vi "Questao1VF_Ulisses.vi"() -> ()   [LabVIEW 2019]
uses:
  <vilib>/measure/matone.llb/Extract Multiple Tone Information 1 Chan.vi
  <vilib>/measure/NI_MAPro.lvlib
panel:
  out "Atende?":bool
  out "DHT(%)":dbl
  out "Fundamental":dbl
  out "Raiz":dbl
  out "Soma Quadratica":dbl
  in  "stop":bool
  in  "LIGAR":bool
  in  "file path":path=path "C:/lista2.tdms"
  out "ONDA COMPLETA":waveform(dbl)(graph)
  out "informação das ondas":T1(array[cluster]) {"detected phase (deg)" format="%_6g"; "detected amplitude" format="%_6p"; "detected frequency" format="%_6p"}
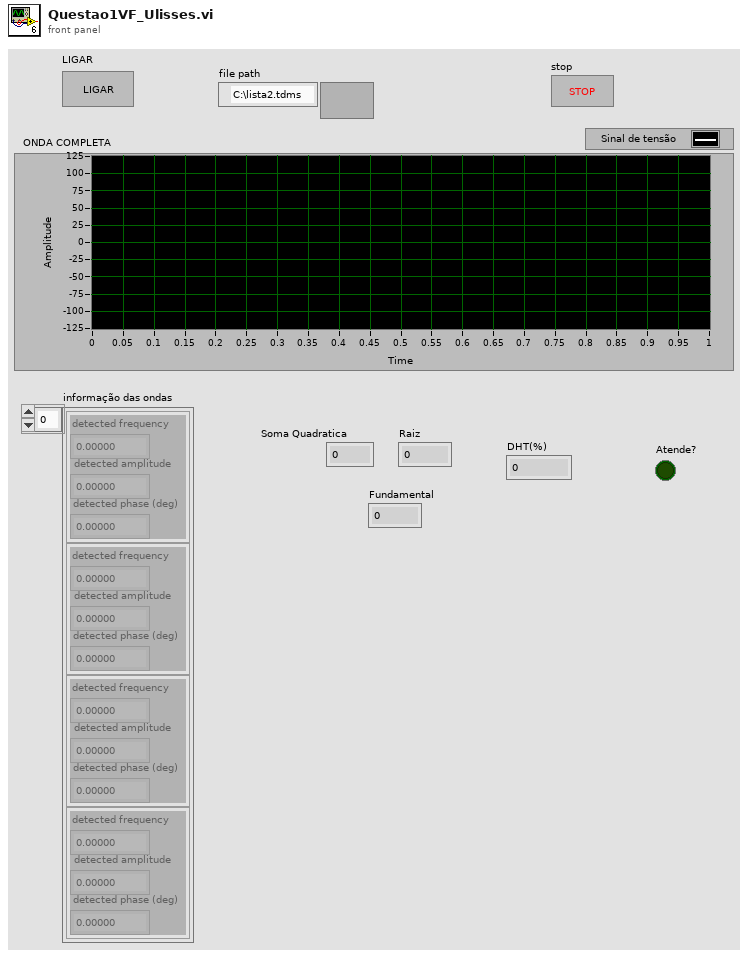
[diagram p1: front panel]
types:
  T1 = cluster{"detected frequency":dbl, "detected amplitude":dbl, "detected phase (deg)":dbl}[]
  T2 = cluster{"detected frequency":dbl, "detected amplitude":dbl, "detected phase (deg)":dbl}
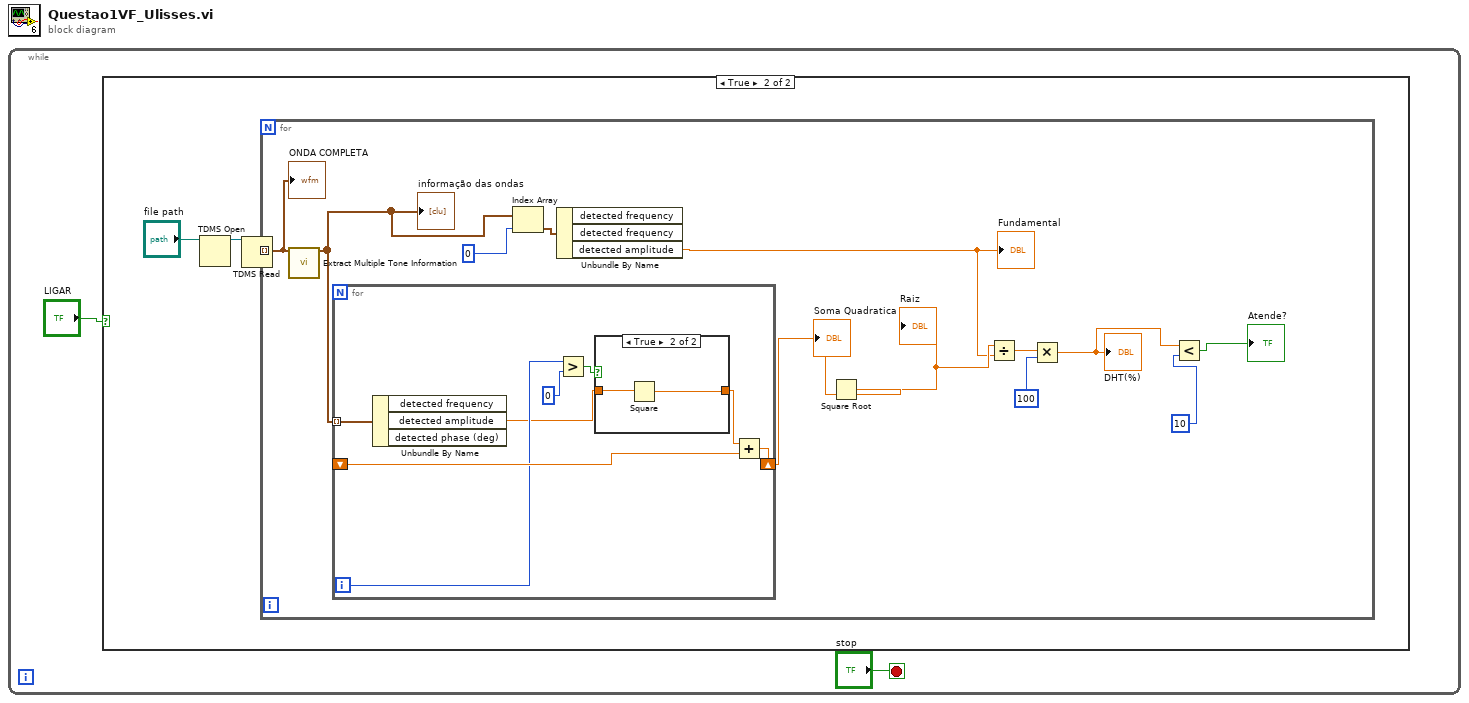
[diagram p0: block diagram]
diagram:
  n1 = while {
    stop <- "stop" stop-if-true
    n2 = case shown="True" "LIGAR" {
      frame False {
      }
      frame True {
        n3 = TDMS Open(11:"file path") -> (3:w4:refnum<k34>)  [unwired: 6 in, 1 out]
        n4 = TDMS Read(0:w4) -> (10:w3:waveform(dbl)[])  [unwired: 7 in, 5 out]
        n5 = for {
          tunnel: w3 -> [w17] mode=indexing
          n6 = call-poly <vilib>:"Extract Multiple Tone Information.vi"("time signal in"=w17) -> ("multiple tone information"=w14:T1)  [unwired: 12 in, 2 out]
          "informação das ondas" <- w14
          n7 = for {
            tunnel: w14 -> [w25] mode=indexing
            shift-right: [w24] -> w16
            shift-left: _ -> [w23]
            i -> [w19]
            n8 = Unbundle By Name(w25) -> ("detected amplitude"=w18:dbl)  [unwired: 2 out]
            n9 = Greater?(x=w19, y=0) -> (0:w20:bool)
            n10 = case shown="True" w20 {
              tunnel: [_ w27] -> w22
              tunnel: w18 -> [_ w26]
              frame False {
              }
              frame True {
                n11 = Square(x=w26) -> (x^2=w27:dbl)
              }
            }
            n12 = Add(x=w22, y=w23) -> (x+y=w24:dbl)
          }
          "Soma Quadratica" <- w16
          n13 = Index Array(array=w14, index=0) -> (element=w13:T2)
          n14 = Unbundle By Name(w13) -> ("detected amplitude"=w11:dbl)  [unwired: 2 out]
          "Fundamental" <- w11
          n15 = Square Root(x=w16) -> (sqrt(x)=w12:dbl)
          "Raiz" <- w12
          n16 = Divide(x=w12, y=w11) -> (x/y=w10:dbl)
          n17 = Multiply(x=w10, y=100) -> (x*y=w8:dbl)
          "DHT(%)" <- w8
          n18 = Less?(x=w8, y=10) -> (x < y?=→"Atende?":bool)
          "ONDA COMPLETA" <- w17
        }
      }
    }
  }
